vi "LP_EQ.VI"(0 "Rotation Vectors":dbl[][](array[numeric]) format="%.2f", 7 "Error in":errorcluster) -> (13 "Error out":errorcluster, 14 "Plane Equation":T1 {"Standard Deviation" format="%.6f"; "Z Slope" format="%.6f"; "Y Slope" format="%.6f"; "Offset" format="%.6f"})   [LabVIEW 2013]
uses:
  <vilib>/Analysis/NI_AALPro.lvlib
panel:
  # "LP Equation Fit"
  # "V1.0 Americo A Migliaccio 8-Oct 97"
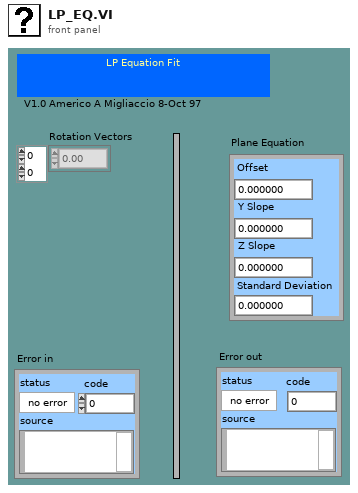
[diagram p1: front panel]
types:
  T1 = cluster{"Offset":dbl, "Y Slope":dbl, "Z Slope":dbl, "Standard Deviation":dbl}
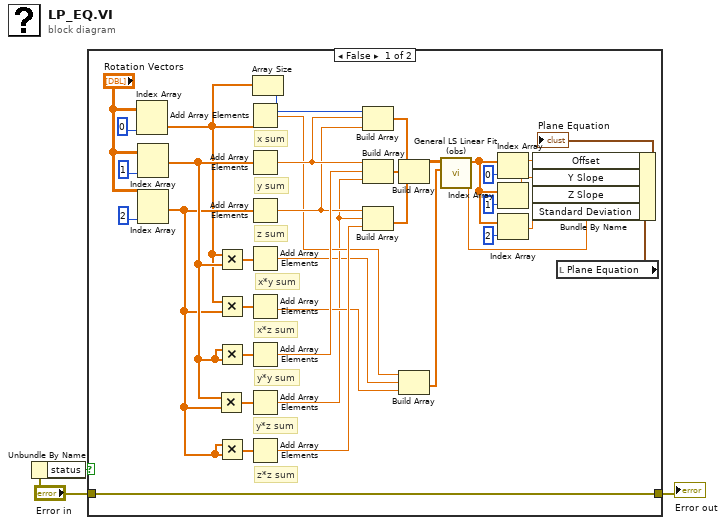
[diagram p0: block diagram]
diagram:
  n1 = Unbundle By Name("Error in") -> ("status"=w1:bool)
  n2 = case shown="False" w1 {
    tunnel: [w7 w41] -> w2
    tunnel: "Error in" -> [w7 w41]
    frame False {
      # "z*z sum"
      # "y*z sum"
      # "y*y sum"
      # "x*z sum"
      # "x*y sum"
      # "z sum"
      # "y sum"
      # "x sum"
      n3 = Index Array(array="Rotation Vectors", index (col)=0) -> (element=w32:dbl[])  [unwired: 1 in]
      n4 = Index Array(array="Rotation Vectors", index (col)=1) -> (element=w34:dbl[])  [unwired: 1 in]
      n5 = Index Array(array="Rotation Vectors", index (col)=2) -> (element=w33:dbl[])  [unwired: 1 in]
      n6 = Multiply(x=w34, y=w33) -> (x*y=w36:dbl[])
      n7 = Multiply(x=w32, y=w34) -> (x*y=w39:dbl[])
      n8 = Multiply(x=w32, y=w33) -> (x*y=w38:dbl[])
      n9 = Multiply(x=w34, y=w34) -> (x*y=w37:dbl[])
      n10 = Multiply(x=w33, y=w33) -> (x*y=w35:dbl[])
      n11 = Add Array Elements(numeric array=w32) -> (sum=w26:dbl)
      n12 = Add Array Elements(numeric array=w34) -> (sum=w30:dbl)
      n13 = Add Array Elements(numeric array=w33) -> (sum=w28:dbl)
      n14 = Add Array Elements(numeric array=w39) -> (sum=w23:dbl)
      n15 = Add Array Elements(numeric array=w38) -> (sum=w25:dbl)
      n16 = Add Array Elements(numeric array=w37) -> (sum=w29:dbl)
      n17 = Add Array Elements(numeric array=w36) -> (sum=w24:dbl)
      n18 = Add Array Elements(numeric array=w35) -> (sum=w27:dbl)
      n19 = Array Size(array=w32) -> (size(s)=w31:i32)
      n20 = Build Array(w31, w30, w28) -> (w22:dbl[])
      n21 = Build Array(w30, w29, w24) -> (w21:dbl[])
      n22 = Build Array(w28, w24, w27) -> (w20:dbl[])
      n23 = Build Array(w22, w21, w20) -> (w19:dbl[][])
      n24 = Build Array(w26, w23, w25) -> (w18:dbl[])
      n25 = call <vilib>:"General LS Linear Fit (obs).vi"("H"=w19, "Y"=w18) -> ("Coefficients"=w14:dbl[], "mse"=w9:dbl)  [unwired: 3 in, 3 out]
      n26 = Index Array(array=w14, index=0) -> (element=w12:dbl)
      n27 = Index Array(array=w14, index=1) -> (element=w11:dbl)
      n28 = Index Array(array=w14, index=2) -> (element=w10:dbl)
      n29 = local read "Plane Equation"() -> (w13:T1)
      n30 = Bundle By Name(cluster=w13, "Offset"=w12, "Y Slope"=w11, "Z Slope"=w10, "Standard Deviation"=w9) -> (→"Plane Equation":T1)
    }
    frame True {
    }
  }
  "Error out" <- w2
